vi "Keypress Global.vi"() -> ()   [LabVIEW 2014]
panel:
  in  "Keypress":enum16{"Right", "Down", "Up", "Left"}(ring)
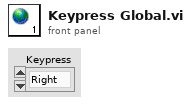
[diagram p1: front panel]
diagram:
